vi "LoggerRef Set.vi"(8 "Logger Error In (no error)":errorcluster, 10 "Logger Ref Name":string, 11 "LoggerRef In":T1) -> (0 "Logger Error Out":errorcluster, 3 "LoggerRef Out":T1)   [LabVIEW 2014]
uses:
  LoggerRef.ctl
  <vilib>/Rock Robotics/WPI/Utilities/Refnum Registry Operation.ctl
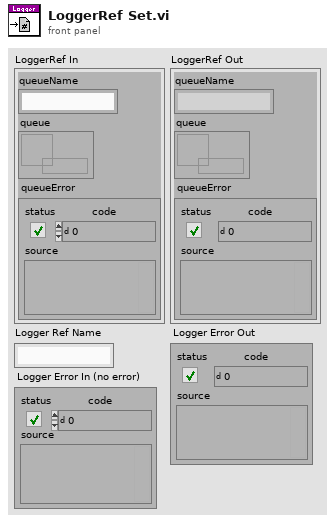
[diagram p1: front panel]
types:
  T1 = typedef "LoggerRef.ctl" = cluster{"queueName":string, "queue":refnum<queue>, "queueError":errorcluster}
  T2 = typedef "Refnum Registry Operation.ctl" = enum16{"set", "get", "delete", "get all names", "read name"}
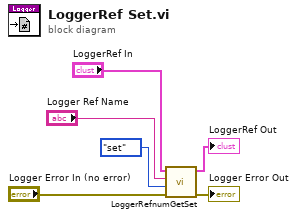
[diagram p0: block diagram]
diagram:
  n1 = call "LoggerRefnumGetSet.vi"("Logger Error In (no error)"="Logger Error In (no error)", "menu"=Refnum_Registry_Operation."set", "Logger Ref Name"="Logger Ref Name", "LoggerRef In"="LoggerRef In") -> ("Logger Error Out"=→"Logger Error Out":errorcluster, "LoggerRef 2 Out"=→"LoggerRef Out":T1)  [unwired: 5 in, 1 out]
